vi "SmartMotor Chain Close.vi"() -> ()   [LabVIEW 2017, in "SmartMotor.lvclass"]
uses:
  SmartMotor.lvclass
panel:
  out "error out":errorcluster
  in  "error in (no error)":errorcluster
  in  "SmartMotor Chain VISA Resource":refnum<visa-resource-name>
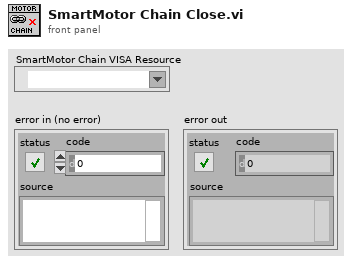
[diagram p1: front panel]
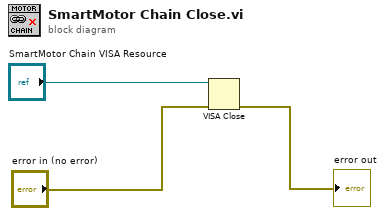
[diagram p0: block diagram]
diagram:
  n1 = VISA Close(VISA resource name="SmartMotor Chain VISA Resource", error in (no error)="error in (no error)") -> (error out=→"error out":errorcluster)
